vi "d-flip-flop.vi"(11 "T":bool) -> (0 "!Q":bool, 3 "Q":bool)   [LabVIEW 2021]
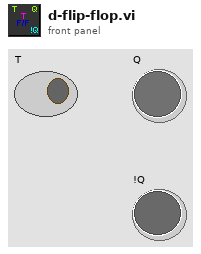
[diagram p1: front panel]
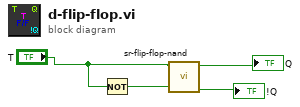
[diagram p0: block diagram]
diagram:
  n1 = Not(x="T") -> (.not. x?=w1:bool)
  n2 = call "sr-flip-flop-nand.vi"("Reset"=w1, "Set"="T") -> ("!Q"=→"!Q":bool, "Q"=→"Q":bool)  [unwired: 8 in]
